vi "(auto) Get State (SubVI).vi"(8 "Dots in total":i32, 9 "States in total":i32, 10 "CurDot":T1(ring), 11 "Dots of States":i32[][](array[numeric])) -> (3 "(auto) States":T1(ring))   [LabVIEW 2017]
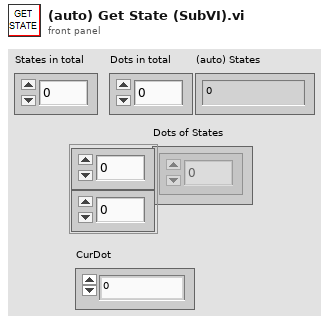
[diagram p1: front panel]
types:
  T1 = enum16{"0", "1", "2", "3", "4", "5", "6", "7", "8", "9", "10", "11", "12", "13", "14", "15", "16", "17", "18", "19", "20", "21", "22", "23", "24", "25", "26", "27", "28", "29", "30", "31", "32", "33", "34", "35"}
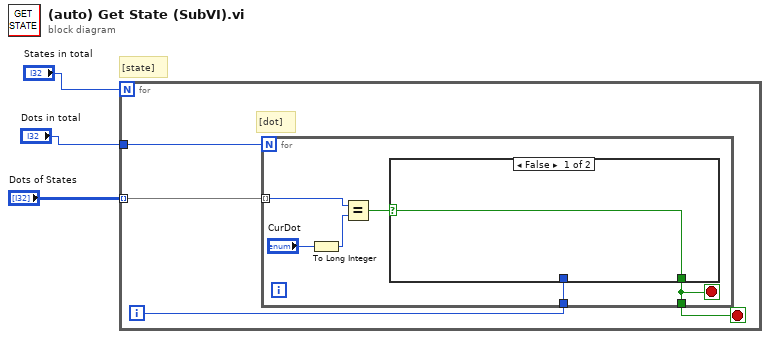
[diagram p0: block diagram]
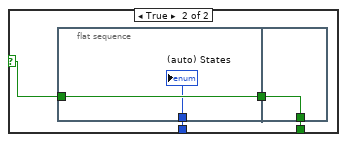
[diagram p2: hidden frame]
diagram:
  # "[state]"
  n1 = for {
    N: "States in total" -> [_]
    tunnel: "Dots in total" -> [w7]
    tunnel: "Dots of States" -> [w6] mode=indexing
    i -> [w5]
    stop <- w4 stop-if-true
    # "[dot]"
    n2 = for {
      N: w7 -> [_]
      tunnel: w6 -> [w13] mode=indexing
      tunnel: w5 -> [w9]
      tunnel: [w8] -> w4
      stop <- w8 stop-if-true
      n3 = To Long Integer(number="CurDot") -> (32bit integer=w11:i32)
      n4 = Equal?(x=w13, y=w11) -> (x = y?=w10:bool)
      n5 = case shown="False" w10 {
        selector: w10 -> [w14 w18]
        tunnel: w9 -> [_ w16]
        tunnel: [w14 w15] -> w8
        frame False {
        }
        frame True {
          n6 = flat-sequence {
            tunnel: w18 -> [w20]
            tunnel: [w20] -> w17
            tunnel: w16 -> [w19]
            tunnel: w17 -> [w21]
            tunnel: [w21] -> w15
            frame #0 {
              "(auto) States" <- w19
            }
            frame #1 {
            }
          }
        }
      }
    }
  }
